vi "plant model(subVI).vi"(4 "dt (s)":dbl=-1.0 format="%.3f", 6 "reinitialize? (F)":bool, 7 "output saturation range":cluster{"output high":dbl, "output low":dbl}={"output high"=inf, "output low"=-inf}, 9 "process parameters":T1={"static gain"=2.5, "lag (s)"=18.0, "deadtime (s)"=0.001, "load"=30.0, "deadband"=2.0, "sensor noise"=0.25, "initial PV"=0.0, "plant noise"=0.0} {"plant noise" format="%.2f"; "initial PV" format="%.2f"; "sensor noise" format="%.2f"; "lag (s)" format="%.2f"; "deadtime (s)" format="%.2f"; "deadband" format="%.1f"; "load" format="%.2f"; "static gain" format="%.2f"}, 10 "Plant Input":dbl format="%.2f", 11 "Integrator ?":bool) -> (3 "Plant Output":dbl format="%.2f")   [LabVIEW 2021]
uses:
  <vilib>/addons/control/pid/pid.llb/PID Lead-Lag (DBL).vi
  <vilib>/addons/control/pid/NI_PID_pid.lvlib
  <vilib>/addons/control/advanced/NI_AdvCtrl_nonlinear.lvlib
panel:
  out "dt out (s)":dbl format="%.3f"
  out "dt (s) out":dbl
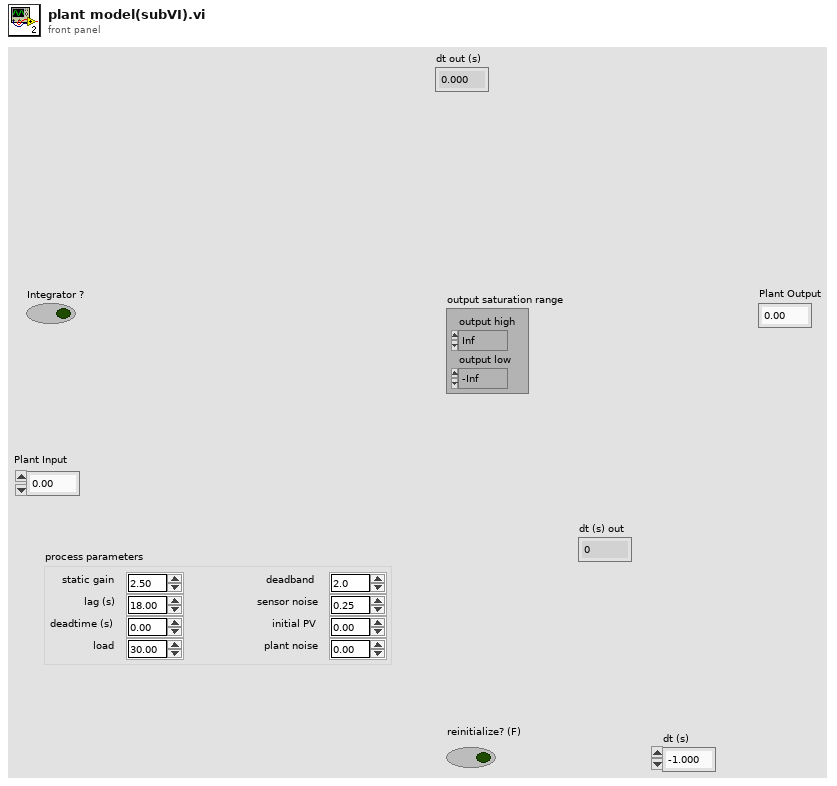
[diagram p1: front panel]
types:
  T1 = cluster{"static gain":dbl, "lag (s)":dbl, "deadtime (s)":dbl, "load":dbl, "deadband":dbl, "sensor noise":dbl, "initial PV":dbl, "plant noise":dbl}
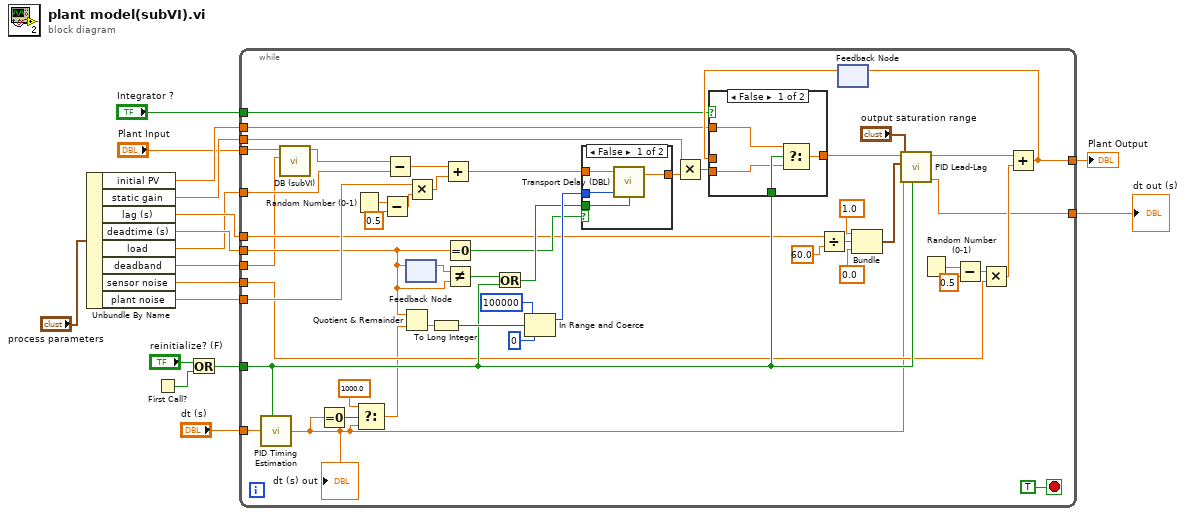
[diagram p0: block diagram]
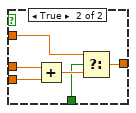
[diagram p3: hidden frame]
diagram:
  n1 = Unbundle By Name("process parameters") -> ("initial PV"=w17:dbl, "static gain"=w13:dbl, "lag (s)"=w15:dbl, "deadtime (s)"=w12:dbl, "load"=w9:dbl, "deadband"=w10:dbl, "sensor noise"=w16:dbl, "plant noise"=w8:dbl)
  n2 = First Call?() -> (First Call?: T/F=w3:bool)
  n3 = Or(x="reinitialize? (F)", y=w3) -> (x .or. y?=w4:bool)
  n4 = while {
    tunnel: w4 -> [w35]
    tunnel: "dt (s)" -> [w36]
    tunnel: [w51] -> w6
    tunnel: w8 -> [w33]
    tunnel: w9 -> [w32]
    tunnel: w10 -> [w19]
    tunnel: "Plant Input" -> [w20]
    tunnel: w12 -> [w25]
    tunnel: w13 -> [w31]
    tunnel: "Integrator ?" -> [w30]
    tunnel: w15 -> [w22]
    tunnel: w16 -> [w29]
    tunnel: w17 -> [w23]
    tunnel: [w18] -> w1
    stop <- TRUE stop-if-true
    n5 = call <vilib>:"PID Timing Estimation.vi"("Initialize?"=w35, "dt (s) in"=w36) -> ("dt (s) out"=w28:dbl)  [unwired: 7 in]
    "dt (s) out" <- w28
    n6 = call "DB (subVI).vi"("deadband (%)"=w19, "requested pos. (%)"=w20) -> ("actual pos. (%)"=w21:dbl)  [unwired: 9 in]
    n7 = Equal To 0?(x=w28) -> (x = 0?=w38:bool)
    n8 = Random Number (0-1)() -> (number: 0 to 1=w65:dbl)
    n9 = Select(t=1000.0, s=w38, f=w28) -> (s? t:f=w26:dbl)
    n10 = Subtract(x=w65, y=0.5) -> (x-y=w34:dbl)
    n11 = Subtract(x=w21, y=w32) -> (x-y=w47:dbl)
    n12 = Quotient & Remainder(x=w25, y=w26) -> (floor(x/y)=w53:dbl)  [unwired: 1 out]
    n13 = feedback-in #1(w25) -> ()
    n14 = feedback #1() -> (w44:dbl)  [unwired: 1 in]
    n15 = Multiply(x=w33, y=w34) -> (x*y=w67:dbl)
    n16 = To Long Integer(number=w53) -> (32bit integer=w42:i32)
    n17 = Add(x=w47, y=w67) -> (x+y=w46:dbl)
    n18 = Equal To 0?(x=w25) -> (x = 0?=w24:bool)
    n19 = Not Equal?(x=w44, y=w25) -> (x != y?=w43:bool)
    n20 = Or(x=w43, y=w35) -> (x .or. y?=w27:bool)
    n21 = In Range and Coerce(upper limit=100000, x=w42, lower limit=0) -> (coerced(x)=w39:i32)  [unwired: 1 out]
    n22 = case shown="False" w24 {
      tunnel: [w71 w72] -> w52
      tunnel: w46 -> [w70 w72]
      tunnel: w39 -> [w69 _]
      tunnel: w27 -> [w68 _]
      frame False {
        n23 = call <vilib>:"Transport Delay (DBL).vi"("initialize"=w68, "delay"=w69, "input point"=w70) -> ("output point"=w71:dbl)  [unwired: 2 in]
      }
      frame True {
      }
    }
    n24 = Multiply(x=w31, y=w52) -> (x*y=w45:dbl)
    n25 = Divide(x=w22, y=60.0) -> (x/y=w49:dbl)
    n26 = feedback #2() -> (w59:dbl)  [unwired: 1 in]
    n27 = case shown="False" w30 {
      tunnel: w45 -> [w75 w82]
      tunnel: [w74 w80] -> w62
      tunnel: w23 -> [w73 w79]
      tunnel: w59 -> [_ w78]
      tunnel: w35 -> [w76 w77]
      frame False {
        n28 = Select(t=w73, s=w76, f=w75) -> (s? t:f=w74:dbl)
      }
      frame True {
        n29 = Add(x=w78, y=w82) -> (x+y=w81:dbl)
        n30 = Select(t=w79, s=w77, f=w81) -> (s? t:f=w80:dbl)
      }
    }
    n31 = Bundle(1.0, w49, 0.0) -> (w60:cluster{dbl, dbl, dbl})  [unwired: 1 in]
    n32 = call-poly <vilib>:"PID Lead-Lag.vi"("reinitialize? (F)"=w35, "dt (s)"=w28, "output range"="output saturation range", "tuning parameters"=w60, "input"=w62) -> ("dt out (s)"=w18:dbl, "output"=w55:dbl)  [unwired: 3 in]
    n33 = Random Number (0-1)() -> (number: 0 to 1=w58:dbl)
    n34 = Subtract(x=w58, y=0.5) -> (x-y=w57:dbl)
    n35 = Multiply(x=w57, y=w29) -> (x*y=w54:dbl)
    n36 = Add(x=w55, y=w54) -> (x+y=w51:dbl)
    n37 = feedback-in #2(w51) -> ()
  }
  "Plant Output" <- w6
  "dt out (s)" <- w1
